vi "UDP2in (SubVI).vi"(8 "error in (no error)":errorcluster, 11 "Queue in":refnum<queue>) -> (0 "error out":errorcluster)   [LabVIEW 2017]
uses:
  Control_EU/DataCluster.ctl
  Control_EU/UNDT_ClusterPackRevers (Type).ctl
  Global_SNK3_HF.vi
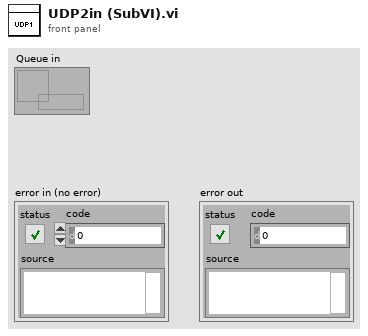
[diagram p1: front panel]
types:
  T1 = cluster{"Packet number":u32, "Reserv":u8, "Packet version":u8, "Packet size":u16}
  T2 = typedef "OptionPACK5.ctl" = cluster{"MagicWordStr":string, "Header size":u32, "Проверка CRC8":bool, "Проверка конца пакета":bool, "GainCompens":bool, "Неотбрасывать BadEnd пакеты":bool, "Неотбрасывать BadCRC пакеты":bool, "Привести к 1":bool, "GainCoef":bool, "K_scale":dbl, "ScaleOrdinate":enum16{"Отсчеты АЦП (±32767)", "Проценты", "Вольты", "дБмкВ (отн. 1 мкВ)", "Отсчеты АЦП (±1)"}}
  T3 = typedef "DataCluster.ctl" = cluster{"UNDT_Cluster":T4, "UNDT_Cluster_Data":dbl[]}
  T4 = typedef "UNDT_ClusterPackRevers (Type).ctl" = cluster{"PacketCounter":u32, "Gain Coeff":sgl, "SamplingInterval":sgl, "Lose Packet":u32, "EncodersParam2":u64, "EncodersParam1":u64, "Reserve 1":u8, "Mux TX/RX":u8, "ScanDelay":u16, "CRC 8":u8, "ScanDuration":u16, "N chanel":u8, "GlobalTime2":u32, "GlobalTime1":u32, "N tick":u8, "Ncycle":u16, "FrameFormatVersion":u8, "MagicWord":u32, "Overload":bool}
  T5 = typedef "Status_pack5.ctl" = cluster{"CRC8Good":bool, "PackEndGood":bool, "MWFind":bool, "PackToSmall":bool, "offset":i32}
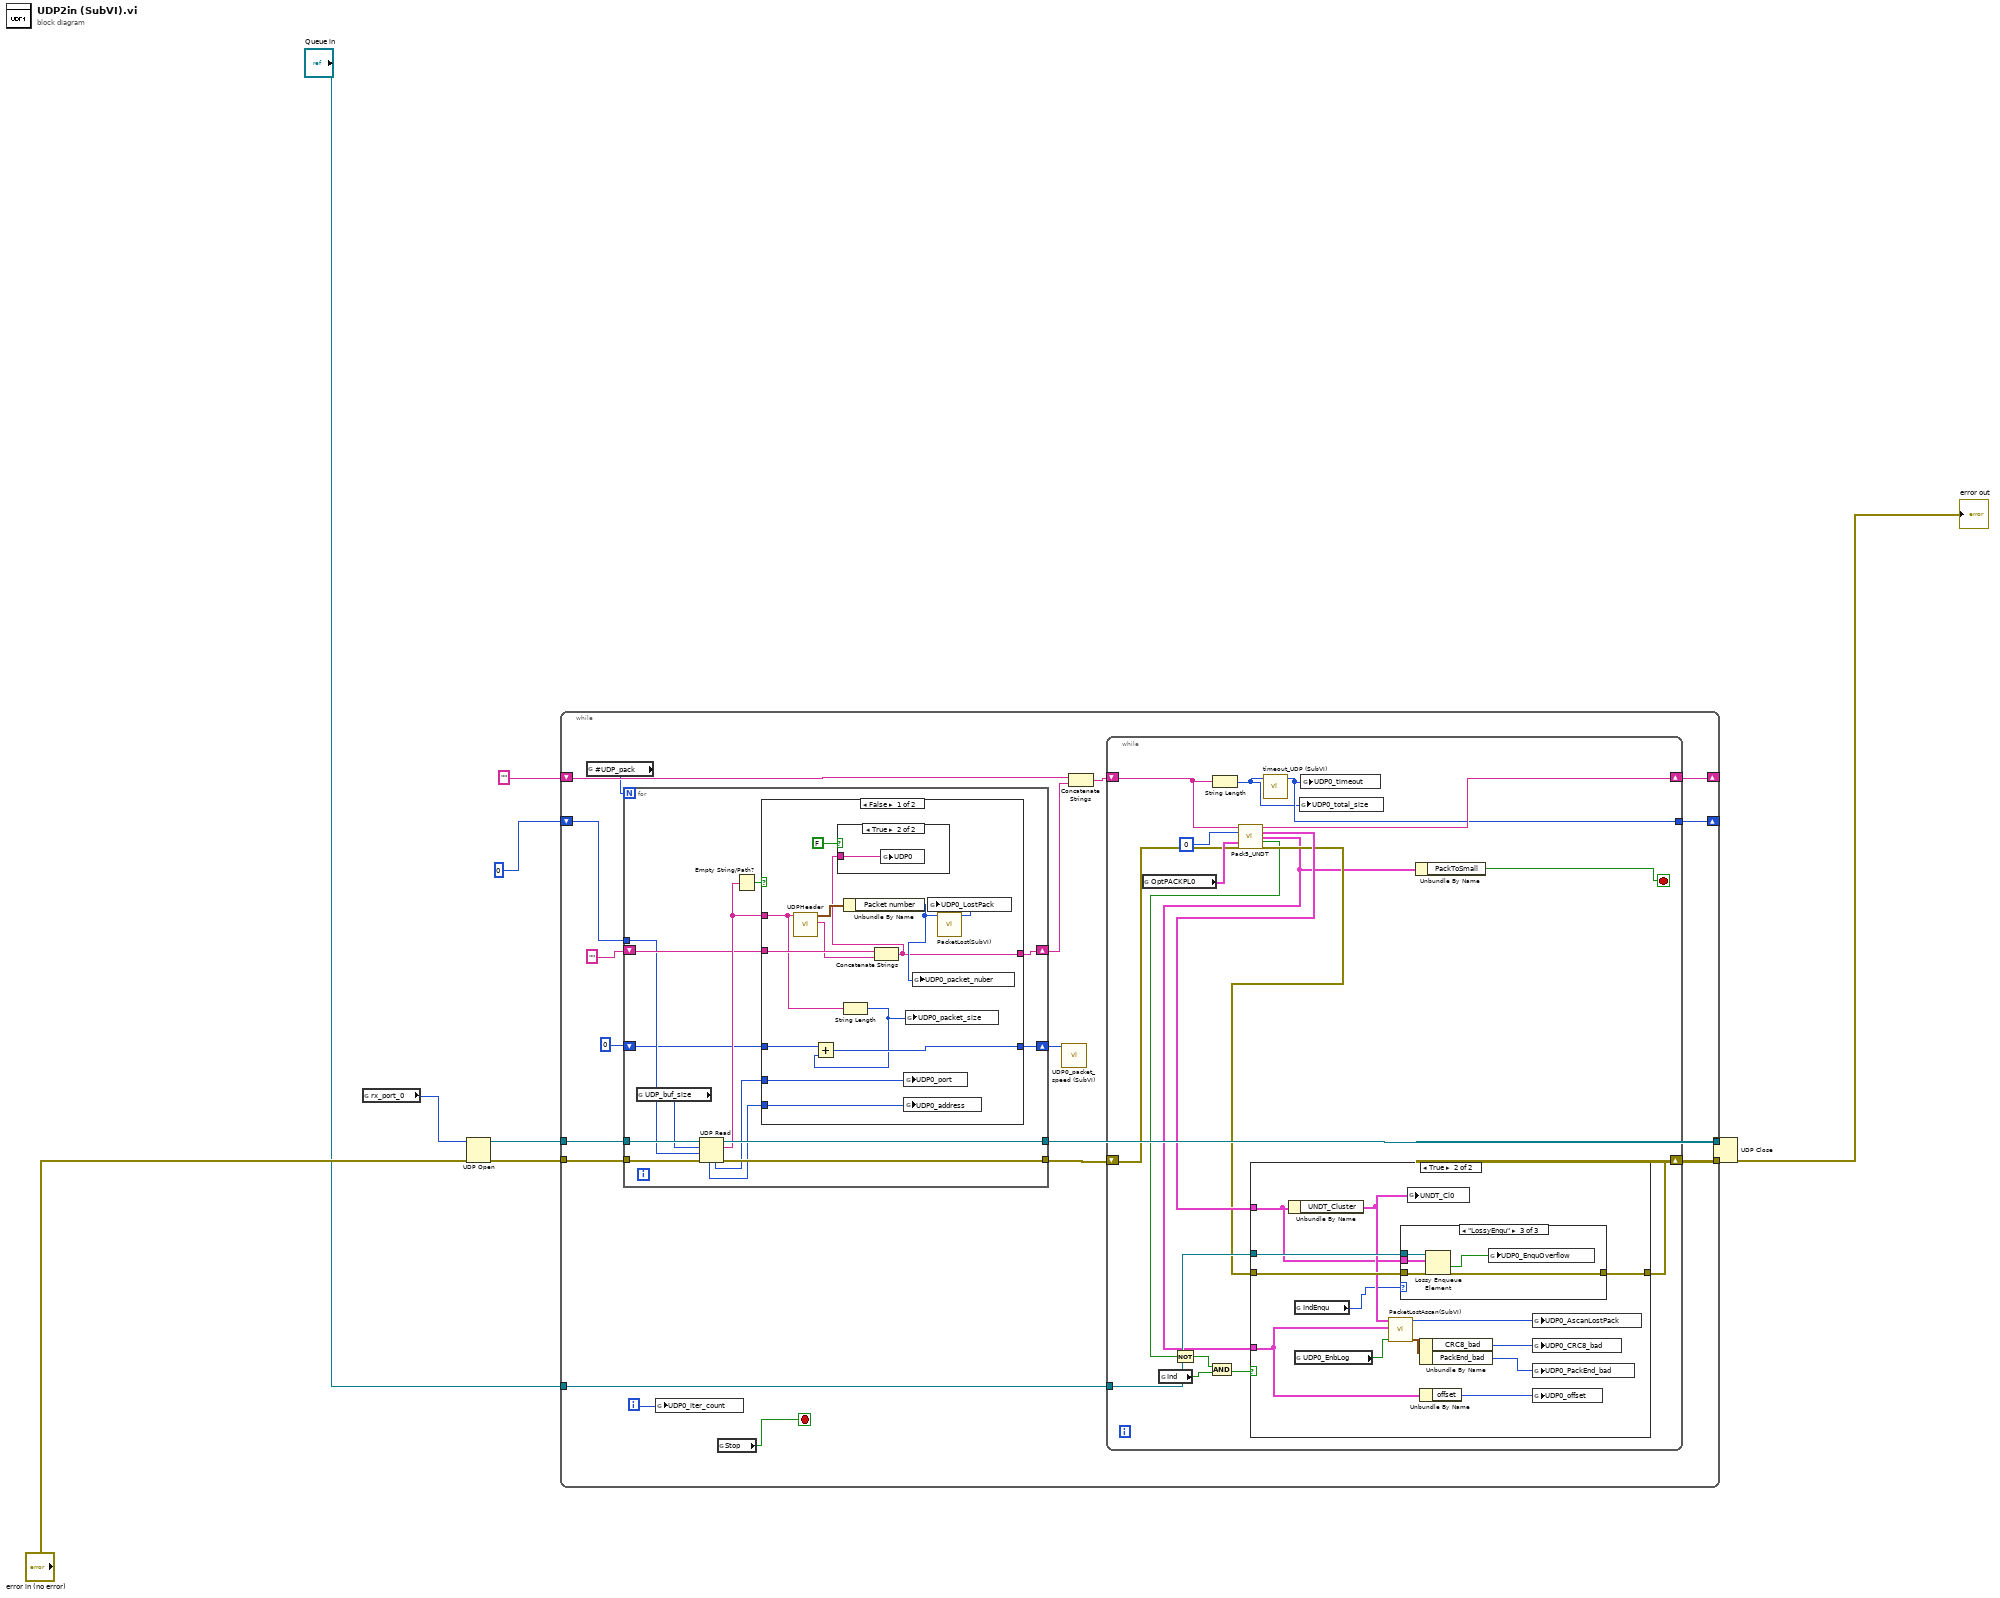
[diagram p0: block diagram]
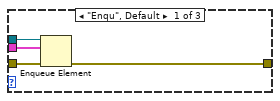
[diagram p3: hidden frame]
diagram:
  n1 = global read "Global_SNK3_HF.vi" "rx_port_0"() -> (w1:u16)
  n2 = UDP Open(8:"error in (no error)", 11:w1) -> (port=w4:refnum<k16>, 0:w5:errorcluster)  [unwired: 3 in, 1 out]
  n3 = while {
    tunnel: w5 -> [w26]
    tunnel: [w14] -> w3
    tunnel: w4 -> [w27]
    tunnel: [w28] -> w2
    shift-right: [w22] -> _
    shift-left: "" ("data out") -> [w23]
    tunnel: "Queue in" -> [w25]
    shift-right: [w18] -> _
    shift-left: 0 ("t") -> [w20]
    i -> [w17]
    stop <- w16 stop-if-true
    n4 = global read "Global_SNK3_HF.vi" "#UDP_pack"() -> (w19:u32)
    n5 = for {
      N: w19 -> [_]
      tunnel: w27 -> [w82]
      tunnel: [w83] -> w28
      tunnel: w26 -> [w81]
      tunnel: [w80] -> w15
      shift-right: [w76] -> w13
      shift-left: "" -> [w77]
      tunnel: w20 -> [w75]
      shift-right: [w71] -> w11
      shift-left: 0 -> [w70]
      n6 = global read "Global_SNK3_HF.vi" "UDP_buf_size"() -> (w74:i32)
      n7 = UDP Read(connection ID=w82, max size (548)=w74, timeout ms (25000)=w75, 8:w81) -> (data out=w79:string, error out=w80:errorcluster, 3:w83:refnum<k16>, 4:w73:u16, 6:w72:u32)
      n8 = Empty String/Path?(string/path=w79) -> (empty?=w78:bool)
      n9 = case shown="False" w78 {
        tunnel: w79 -> [w87 _]
        tunnel: w77 -> [w96 w99]
        tunnel: [w89 w99] -> w76
        tunnel: w73 -> [w93 _]
        tunnel: w72 -> [w92 _]
        tunnel: [w85 w98] -> w71
        tunnel: w70 -> [w86 w98]
        frame False {
          n10 = call "UDPHeader.vi"("String in"=w87) -> ("String out"=w88:string, "UDP header"=w95:T1)  [unwired: 9 in]
          n11 = Unbundle By Name(w95) -> ("Packet number"=w90:u32)
          n12 = String Length(string=w87) -> (length=w84:i32)
          n13 = Add(x=w86, y=w84) -> (x+y=w85:i32)
          n14 = Concatenate Strings(w96, w88) -> (w89:string)
          n15 = case shown="True" FALSE {
            tunnel: w89 -> [_ w97]
            frame False {
            }
            frame True {
              n16 = global write "Global_SNK3_HF.vi" "UDP0"(w97) -> ()
            }
          }
          n17 = global write "Global_SNK3_HF.vi" "UDP0_port"(w93) -> ()
          n18 = global write "Global_SNK3_HF.vi" "UDP0_address"(w92) -> ()
          n19 = global write "Global_SNK3_HF.vi" "UDP0_packet_size"(w84) -> ()
          n20 = global write "Global_SNK3_HF.vi" "UDP0_packet_nuber"(w90) -> ()
          n21 = call "PacketLost(SubVI).vi"("PacketCounter"=w90) -> ("CountLostPack out"=w94:u32)  [unwired: 8 in, 2 out]
          n22 = global write "Global_SNK3_HF.vi" "UDP0_LostPack"(w94) -> ()
        }
        frame True {
        }
      }
    }
    n23 = global write "Global_SNK3_HF.vi" "UDP0_iter_count"(w17) -> ()
    n24 = global read "Global_SNK3_HF.vi" "Stop"() -> (w16:bool)
    n25 = call "UDP0_packet_speed (SubVI).vi"("Data_size"=w11) -> ()  [unwired: 10 in, 1 out]
    n26 = Concatenate Strings(w23, w13) -> (w21:string)
    n27 = while {
      tunnel: w25 -> [w44]
      tunnel: [w39] -> w18
      shift-right: [w43] -> w22
      shift-left: w21 -> [w42]
      shift-right: [w36] -> w14
      shift-left: w15 -> [w38]
      stop <- w29 stop-if-true
      n28 = global read "Global_SNK3_HF.vi" "OptPACKPL0"() -> (w41:T2)
      n29 = global read "Global_SNK3_HF.vi" "Ind"() -> (w35:bool)
      n30 = String Length(string=w42) -> (length=w31:i32)
      n31 = call "Pack5_UNDT.vi"("data in"=w42, "N tick"=u8 0, "OptionPACK5"=w41, "error in"=w38) -> ("data out"=w43:string, "output cluster 2"=w40:T3, "Status"=w30:T5, "PackToSmall"=w34:bool, "error out"=w37:errorcluster)  [unwired: 7 in]
      n32 = Not(x=w34) -> (.not. x?=w33:bool)
      n33 = And(x=w33, y=w35) -> (x .and. y?=w32:bool)
      n34 = case shown="True" w32 {
        tunnel: w44 -> [_ w59]
        tunnel: w37 -> [w46 w58]
        tunnel: [w46 w57] -> w36
        tunnel: w40 -> [_ w53]
        tunnel: w30 -> [_ w54]
        frame False {
        }
        frame True {
          n35 = Unbundle By Name(w53) -> ("UNDT_Cluster"=w56:T4)
          n36 = global read "Global_SNK3_HF.vi" "IndEnqu"() -> (w48:enum16{"NoEnqu", "LossyEnqu", "Enqu"})
          n37 = global read "Global_SNK3_HF.vi" "UDP0_EnbLog"() -> (w47:bool)
          n38 = call "PacketLostAscan(SubVI).vi"("Enable log"=w47, "Status"=w54, "UNDT_Cl1"=w56) -> ("Cluster"=w52:cluster{"CRC8_bad":u32, "PackEnd_bad":u32}, "CountLostPack out"=w49:u32)  [unwired: 5 in, 2 out]
          n39 = case shown="\"LossyEnqu\"" w48 {
            tunnel: w59 -> [w61 _ w69]
            tunnel: w58 -> [w63 w64 w68]
            tunnel: [w62 w64 w67] -> w57
            tunnel: w53 -> [w60 _ w66]
            frame "Enqu", Default {
              n40 = Enqueue Element(queue=w61, element=w60, error in (no error)=w63) -> (error out=w62:errorcluster)  [unwired: 1 in, 2 out]
            }
            frame "NoEnqu" {
            }
            frame "LossyEnqu" {
              n41 = Lossy Enqueue Element(queue=w69, element=w66, error in (no error)=w68) -> (overflow?=w65:bool, error out=w67:errorcluster)  [unwired: 2 out]
              n42 = global write "Global_SNK3_HF.vi" "UDP0_EnquOverflow"(w65) -> ()
            }
          }
          n43 = global write "Global_SNK3_HF.vi" "UNDT_Cl0"(w56) -> ()
          n44 = Unbundle By Name(w52) -> ("CRC8_bad"=w50:u32, "PackEnd_bad"=w51:u32)
          n45 = Unbundle By Name(w54) -> ("offset"=w55:i32)
          n46 = global write "Global_SNK3_HF.vi" "UDP0_AscanLostPack"(w49) -> ()
          n47 = global write "Global_SNK3_HF.vi" "UDP0_CRC8_bad"(w50) -> ()
          n48 = global write "Global_SNK3_HF.vi" "UDP0_PackEnd_bad"(w51) -> ()
          n49 = global write "Global_SNK3_HF.vi" "UDP0_offset"(w55) -> ()
        }
      }
      n50 = call "timeout_UDP (SubVI).vi"("length"=w31) -> ("timeout UDP"=w39:i32)  [unwired: 10 in]
      n51 = global write "Global_SNK3_HF.vi" "UDP0_total_size"(w31) -> ()
      n52 = global write "Global_SNK3_HF.vi" "UDP0_timeout"(w39) -> ()
      n53 = Unbundle By Name(w30) -> ("PackToSmall"=w29:bool)
    }
  }
  n54 = UDP Close(connection ID=w2, 8:w3) -> (error out=→"error out":errorcluster)  [unwired: 1 out]
